vi "Create Axis Rails.vi"(8 "error in (no error)":errorcluster, 11 "XRay Axis Rails in":refnum<class "XRay Axis Rails.lvclass">) -> (0 "error out":errorcluster, 3 "XRay Axis Rails out":refnum<class "XRay Axis Rails.lvclass">)   [LabVIEW 2026, in "XRay Axis Rails.lvclass"]
uses:
  XRay Axis Rails.lvclass
  XRay Axis Rails.lvclass/XRay Axis Rails.ctl
  <vilib>/picture/3D Picture Control/Object/Create Object (drawable).vi
  <vilib>/picture/3D Picture Control/NI_3D Picture Control.lvlib
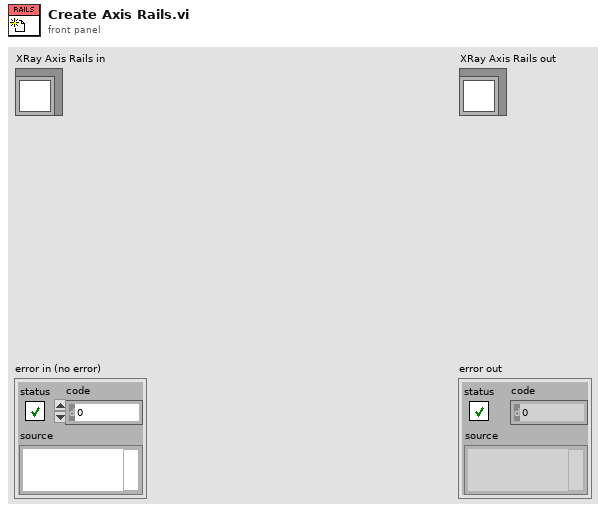
[diagram p1: front panel]
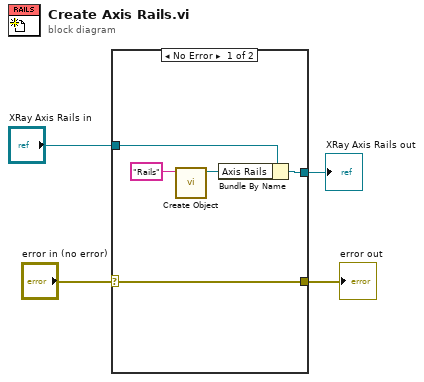
[diagram p0: block diagram]
diagram:
  n1 = case shown="No Error" "error in (no error)" {
    selector: "error in (no error)" -> [w9 w10]
    tunnel: [w9 w10] -> w3
    tunnel: [w7 w11] -> w1
    tunnel: "XRay Axis Rails in" -> [w8 w11]
    frame No Error {
      n2 = call-poly <vilib>:"Create Object.vi"("Name"="Rails") -> ("Scene:New Object"=w5:refnum<vi>)  [unwired: 9 in, 1 out]
      n3 = Bundle By Name(cluster=w8, "Axis Rails"=w5) -> (w7:refnum<class "XRay Axis Rails.lvclass">)
    }
    frame Error {
    }
  }
  "error out" <- w3
  "XRay Axis Rails out" <- w1
